vi "Create Content.vi"(5 "HttpContent in":refnum<class "HttpContent.lvclass">, 6 "timeout_ms":i32, 8 "error in (no error)":errorcluster, 11 "NET_HttpContent":refnum<k24>) -> (0 "error out":errorcluster, 3 "HttpContent out":refnum<class "HttpContent.lvclass">)   [LabVIEW 2018, in "HttpClient_NET.lvlib" / "HttpContent.lvclass"]
uses:
  HttpContent.lvclass
  System.Net.Http
  HttpContent.lvclass/HttpContent.ctl
  Accessors/Write NET_HttpContent.vi
  Accessors/Write timeout_ms.vi
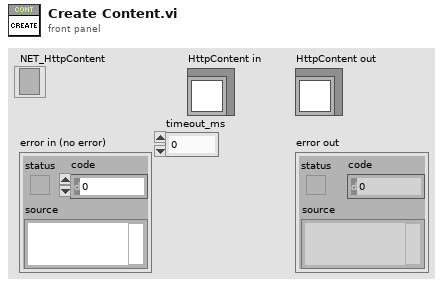
[diagram p1: front panel]
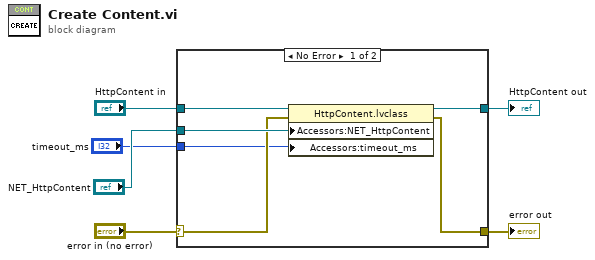
[diagram p0: block diagram]
diagram:
  n1 = case shown="No Error" "error in (no error)" {
    selector: "error in (no error)" -> [w9 w14]
    tunnel: [w8 w14] -> w5
    tunnel: [w11 w13] -> w3
    tunnel: "HttpContent in" -> [w12 w13]
    tunnel: "NET_HttpContent" -> [w10 _]
    tunnel: "timeout_ms" -> [w7 _]
    frame No Error {
      n2 = property class="HttpContent.lvclass"(reference=w12, error in=w9, "Accessors:NET_HttpContent"=w10, "Accessors:timeout_ms"=w7) -> (reference out=w11:refnum<class "HttpContent.lvclass">, error out=w8:errorcluster)
    }
    frame Error {
    }
  }
  "error out" <- w5
  "HttpContent out" <- w3
